vi "PlayerStart.vi"(9 "Default Positions":i16[](array[numeric])=[0], 10 "Filename":string, 11 "NXT":T1={"Hardware"="NXT", "Flattened String"=""}) -> (3 "NXT":T1={"Hardware"="NXT", "Flattened String"=""})   [LabVIEW 2010, in "Player.lvlib"]
uses:
  Player.lvlib
  <vilib>/NXT/Subs/LVHSConnector.ctl
  CLIB/CRef/Interface/CRef Boolean.llb/Boolean CReference.ctl
  CLIB/CThread/Core/CThread Thread Properties.ctl
  CLIB/CThread/XNodes/referencenode/CThread VI Reference.xnode
  CLIB/CThread/XNodes/terminalnode/CThread VI Terminal Node.xnode
  CLIB/CThread/Base/CThread Base - VI Reference.vi
  CLIB/CThread/Base/CThread Base - While Loop.vi
  CLIB/CRef/Interface/CRef Numeric.llb/I32 CReference.ctl
  CLIB/CRef/CRef.lvlib
  CLIB/CThread/CThread.lvlib
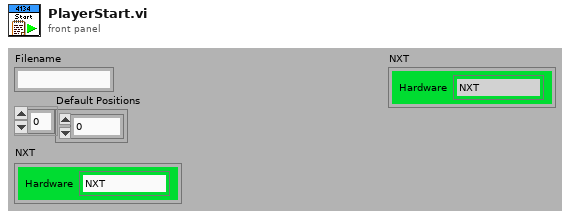
[diagram p1: front panel]
types:
  T1 = typedef "LVHSConnector.ctl" = cluster{"Hardware":string, "Flattened String":string}
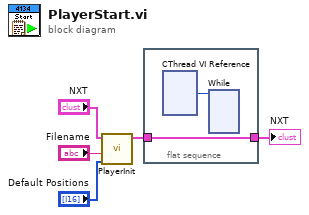
[diagram p0: block diagram]
diagram:
  n1 = call "PlayerInit.vi"("Default Positions"="Default Positions", "Filename"="Filename", "NXT"="NXT") -> ("NXT"=w3:T1)  [unwired: 8 in]
  n2 = flat-sequence {
    tunnel: w3 -> [w6]
    tunnel: [w6] -> w1
    frame #0 {
      n3 = xnode "CThread VI Reference"() -> ("PlayerMain.vi"=w7:i32)
      n4 = xnode "While"("CLIB VI Reference"=w7) -> ()  [unwired: 2 in, 2 out]
    }
  }
  "NXT" <- w1
